vi "Mod_OFDM_Down_Sampling.vi"(0 "input complex waveform":T1={"t0"=0.0, "dt"=1.0, "Y"=[]} {"Y" format="%.3f"; "dt" format="%^.2e"; "t0" format="%.4f"}, 7 "matched filter coefficients":dbl[](array[numeric]) format="%^.2e", 11 "error in (no error)":errorcluster, 12 "Pulse Shaping":T2={"System Filter"={"TX Filter"=enum."Root Raised Cos", "Alpha"=0.5, "filter length"=8}, "Modulation system parameters"={"samples per symbol (16)"=16}, "symbol rate (Hz)"=1.0} {"symbol rate (Hz)" min=1.0 step=1.0 format="%.2p"; "Modulation system parameters"."samples per symbol (16)" step=2; "System Filter"."Alpha" min=0.0 max=1.0 step=0.05 format="%.2f"}, 13 "reset? (T)":bool=TRUE) -> (4 "output complex waveform":T1 {"Y" format="%.3f"; "dt" format="%^.2e"; "t0" format="%.4f"}, 15 "error out":errorcluster)   [LabVIEW 2010]
uses:
  <vilib>/addons/Modulation/Analog/controls/Complex Data Waveform.ctl
  Controls(Type_DEf)/Configure Pulse Shaping.ctl
  <vilib>/addons/Modulation/Digital/General/MT Apply Matched Filter (Generic).vi
  <vilib>/addons/Modulation/Digital/General/MT Align to Ideal Symbols (Generic).vi
panel:
  out "size prior to MF":i32
  out "size post decimation":i32
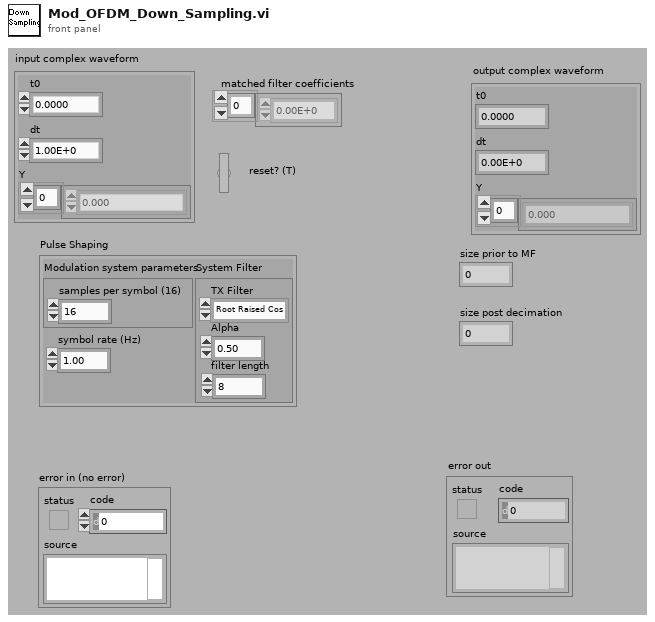
[diagram p1: front panel]
types:
  T1 = typedef "Complex Data Waveform.ctl" = cluster{"t0":dbl, "dt":dbl, "Y":cdb[]}
  T2 = typedef "Configure Pulse Shaping.ctl" = cluster{"System Filter":cluster{"TX Filter":enum16{"none", "Raised Cosine", "Root Raised Cos"}, "Alpha":dbl, "filter length":i32}, "Modulation system parameters":cluster{"samples per symbol (16)":u32}, "symbol rate (Hz)":dbl}
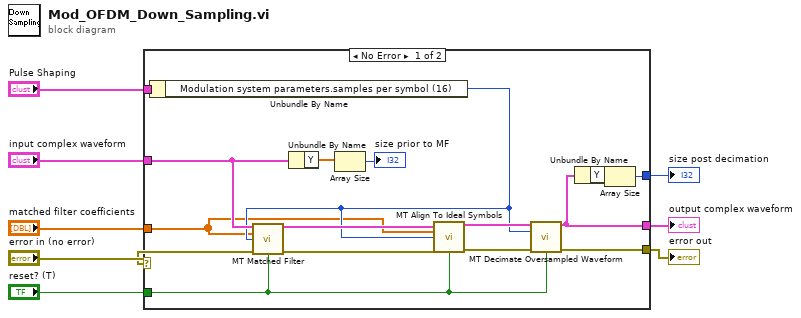
[diagram p0: block diagram]
diagram:
  n1 = case shown="No Error" "error in (no error)" {
    selector: "error in (no error)" -> [w16 w25]
    tunnel: "matched filter coefficients" -> [w10 _]
    tunnel: "reset? (T)" -> [w9 _]
    tunnel: "Pulse Shaping" -> [w24 _]
    tunnel: [w23 w25] -> w5
    tunnel: [w22 _] -> w4
    tunnel: [w20 _] -> w3
    tunnel: "input complex waveform" -> [w17 _]
    frame No Error {
      n2 = Unbundle By Name(w24) -> ("Modulation system parameters.samples per symbol (16)"=w11:u32)
      n3 = call-poly <vilib>:"MT Matched Filter.vi"("input complex waveform"=w17, "matched filter coefficients"=w10, "samples per symbol (16)"=w11, "error in (no error)"=w16, "reset? (T)"=w9) -> ("output complex waveform"=w13:T1, "error out"=w15:errorcluster)  [unwired: 9 in]
      n4 = Unbundle By Name(w17) -> ("Y"=w18:cdb[])
      n5 = Array Size(array=w18) -> (size(s)=→"size prior to MF":i32)
      n6 = call-poly <vilib>:"MT Align To Ideal Symbols.vi"("input complex waveform"=w13, "matched filter coefficients"=w10, "samples per symbol (16)"=w11, "error in (no error)"=w15, "reset? (T)"=w9) -> ("output complex waveform"=w12:T1, "error out"=w14:errorcluster)  [unwired: 8 in, 1 out]
      n7 = call <vilib>:"MT Decimate Oversampled Waveform.vi"("input complex waveform"=w12, "decimation factor"=w11, "error in (no error)"=w14, "reset? (T)"=w9) -> ("output complex waveform"=w20:T1, "error out"=w23:errorcluster)  [unwired: 10 in]
      n8 = Unbundle By Name(w20) -> ("Y"=w21:cdb[])
      n9 = Array Size(array=w21) -> (size(s)=w22:i32)
    }
    frame Error {
    }
  }
  "output complex waveform" <- w3
  "error out" <- w5
  "size post decimation" <- w4
